vi "TwoBallAuton.vi"(11 "Intake Suck at Beginning?":bool) -> ()   [LabVIEW 2013]
uses:
  <vilib>/Rock Robotics/WPI/SafetyOutput/WPI_SafetyOutputConfigMenu.ctl
  <vilib>/Rock Robotics/WPI/Solenoid/WPI_SolenoidValue.ctl
  <vilib>/Rock Robotics/WPI/RobotDrive/WPI_RobotDriveGetSetRefNum.vi
  <vilib>/Rock Robotics/WPI/Solenoid/WPI_SolenoidSetEnum.vi
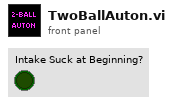
[diagram p1: front panel]
types:
  T1 = typedef "WPI_SafetyOutputConfigMenu.ctl" = enum16{"Enable", "Disable"}
  T2 = typedef "WPI_RobotDriveDevRef.ctl" = cluster{"DevStatus":errorcluster, "Motors[]":T3[], "Square Inputs":bool, "Max Output":dbl, "Isochronous":bool}
  T3 = typedef "WPI_MotorControlDeviceRef.ctl" = cluster{"DeviceStatus":errorcluster, "Type":enum16{"PWM", "CAN"}, "PWM":cluster{"Digital Module":T4, "PWM Channel":T5, "DeadBand":T6}, "CAN":cluster{"Device Number":u8, "Control Mode":T7, "Semaphore":T8, "Max Vout":dbl}, "Invert":bool, "TransformRef":T9, "InvTransformRef":T9}
  T4 = typedef "FPGA_TypedefDigitalModule.ctl" = enum16{"Digital Module 1", "Digital Module 2"}
  T5 = typedef "FPGA_DIOPWMChannel.ctl" = enum8{"PWM 1", "PWM 2", "PWM 3", "PWM 4", "PWM 5", "PWM 6", "PWM 7", "PWM 8", "PWM 9", "PWM 10", "Invalid"}
  T6 = typedef "WPI_PWMDeadband.ctl" = cluster{"Name":string, "maxPositivePwm":i32, "minPositivePwm":i32, "centerPwm":i32, "maxNegativePwm":i32, "minNegativePwm":i32, "angularRange":u16}
  T7 = typedef "WPI_CANJaguar_ControlMode.ctl" = enum8{"Percent VBus", "Current", "Speed", "Position", "Voltage"}
  T8 = typedef "Semaphore RefNum" = refnum<k1>
  T9 = typedef "WPI_PWMTransform_ConPane.ctl" = refnum<vi>
  T10 = typedef "WPI_DigitalInputDevRef.ctl" = cluster{"DevStatus":errorcluster, "DIO Channel":T11, "Digital Module":T4}
  T11 = typedef "FPGA_DIOChannel.ctl" = enum8{"DIO 1", "DIO 2", "DIO 3", "DIO 4", "DIO 5", "DIO 6", "DIO 7", "DIO 8", "DIO 9", "DIO 10", "DIO 11", "DIO 12", "DIO 13", "DIO 14", "Invalid"}
  T12 = typedef "WPI_SolenoidDevRef.ctl" = cluster{"DevStatus":errorcluster, "Solenoid Module":T13, "Forward Solenoid Channel":T14, "Reverse Solenoid Channel":T14}
  T13 = typedef "FPGA_TypedefSolenoidModule.ctl" = enum16{"Solenoid Module 1", "Solenoid Module 2"}
  T14 = typedef "WPI_SolenoidChannel.ctl" = enum8{"Solenoid 1", "Solenoid 2", "Solenoid 3", "Solenoid 4", "Solenoid 5", "Solenoid 6", "Solenoid 7", "Solenoid 8", "Invalid"}
  T15 = typedef "WPI_EncoderDevRef.ctl" = cluster{"DevStatus":errorcluster, "EncoderIndex":T16, "CounterIndex":T17, "DistancePerCount":dbl, "Decoding Type":T18}
  T16 = typedef "FPGA_EncoderIdx.ctl" = enum8{"Enc 0", "Enc 1", "Enc 2", "Enc 3", "Invalid"}
  T17 = typedef "FPGA_CounterCtrSystemIndex.ctl" = enum8{"Ctr 0", "Ctr 1", "Ctr 2", "Ctr 3", "Ctr 4", "Ctr 5", "Ctr 6", "Ctr 7", "Invalid"}
  T18 = typedef "WPI_EncoderType.ctl" = enum16{"1x", "2x", "4x"}
  T19 = typedef "WPI_SolenoidValue.ctl" = enum16{"Off", "On", "Forward", "Reverse"}
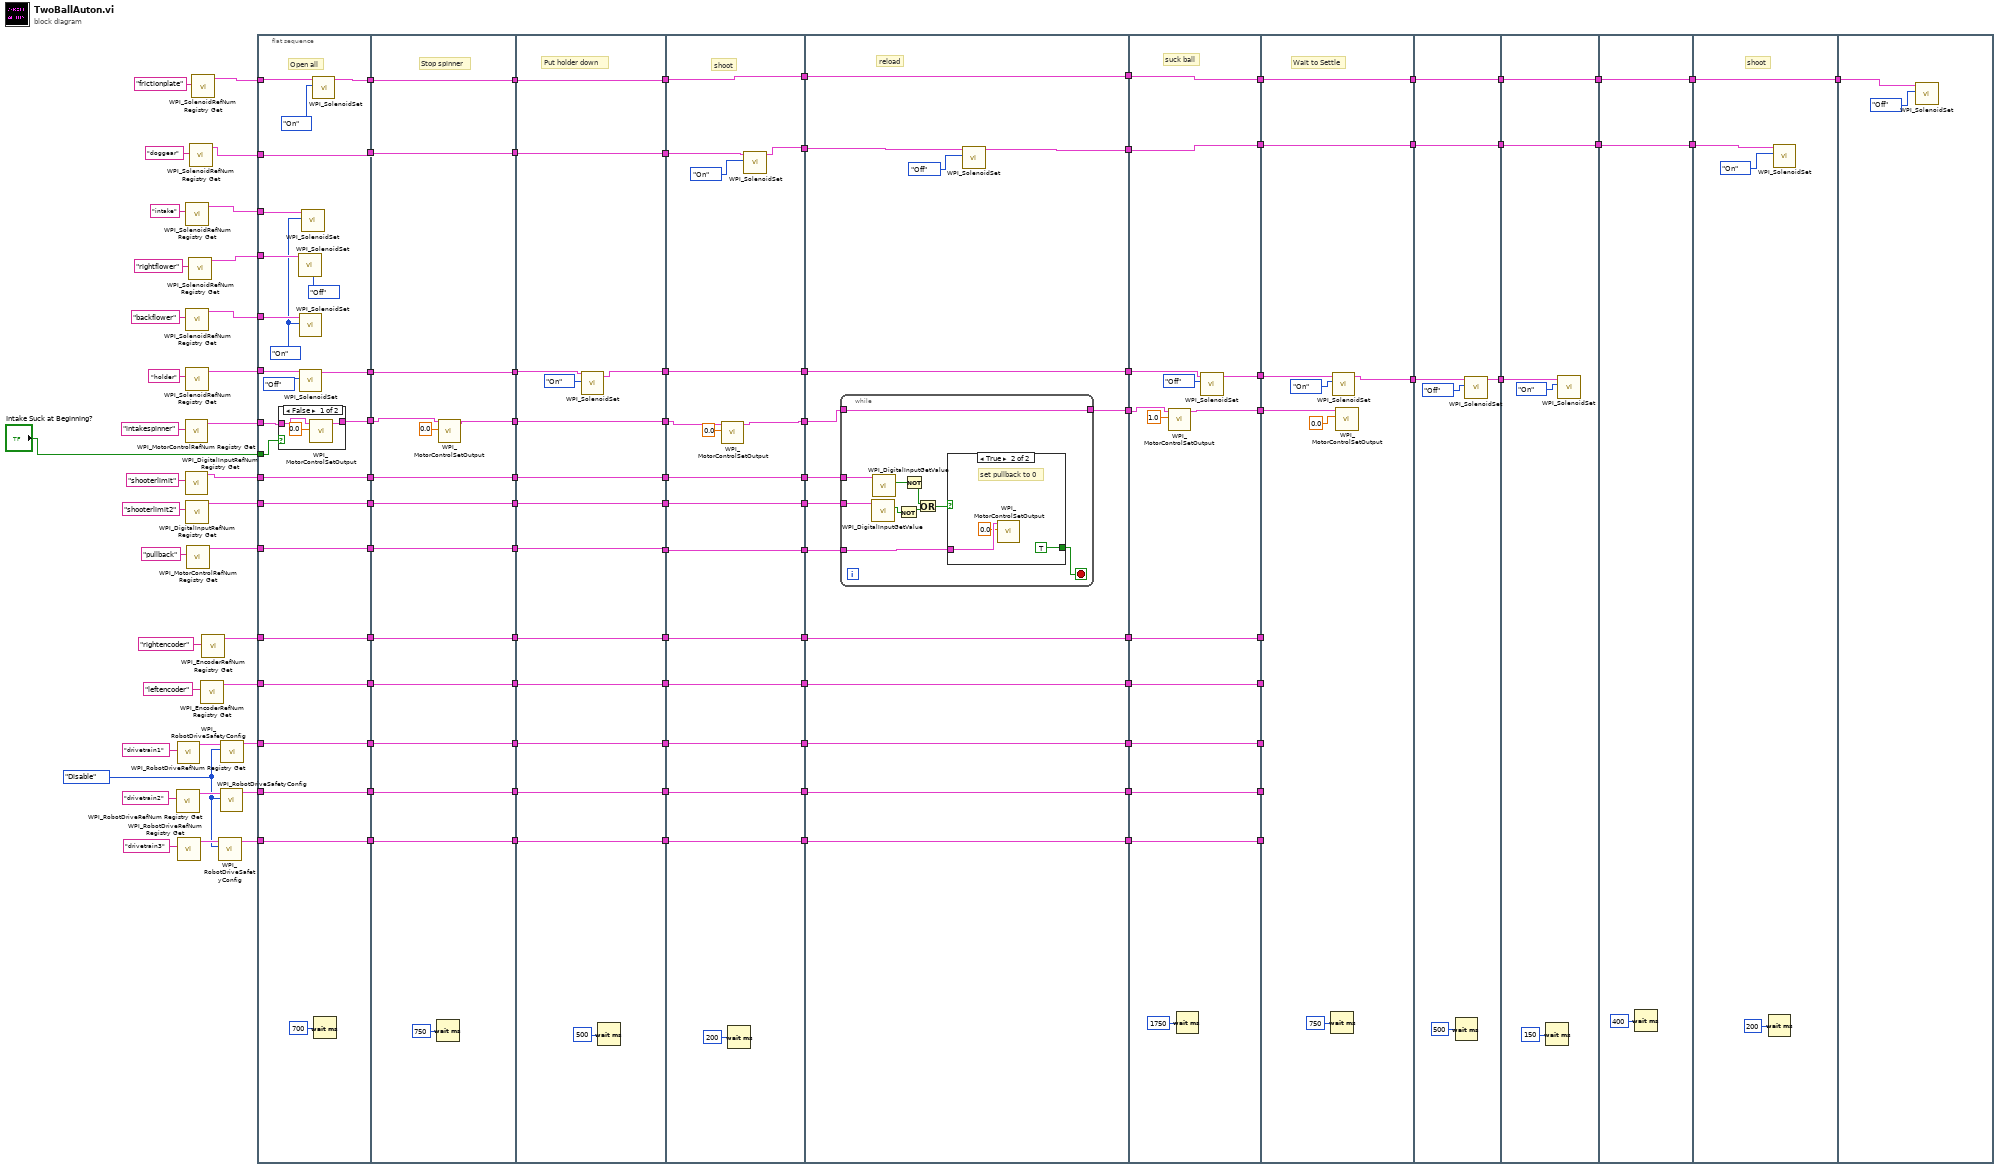
[diagram p0: block diagram]
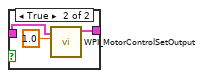
[diagram p2: hidden frame]
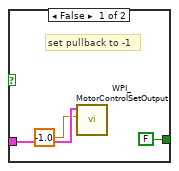
[diagram p3: hidden frame]
diagram:
  w58 = WPI_SafetyOutputConfigMenu."Disable" ("mode")
  n1 = call <vilib>:"WPI_RobotDriveRefNum Registry Get.vi"("refnum name"="drivetrain2") -> ("RobotDriveDevRef"=w60:T2)  [unwired: 9 in, 1 out]
  n2 = call <vilib>:"WPI_RobotDriveRefNum Registry Get.vi"("refnum name"="drivetrain1") -> ("RobotDriveDevRef"=w61:T2)  [unwired: 9 in, 1 out]
  n3 = call <vilib>:"WPI_RobotDriveRefNum Registry Get.vi"("refnum name"="drivetrain3") -> ("RobotDriveDevRef"=w59:T2)  [unwired: 9 in, 1 out]
  n4 = call <vilib>:"WPI_MotorControlRefNum Registry Get.vi"("refnum name"="intakespinner") -> ("MotorControlDevRef"=w71:T3)  [unwired: 9 in, 1 out]
  n5 = call <vilib>:"WPI_DigitalInputRefNum Registry Get.vi"("refnum name"="shooterlimit") -> ("DigitalInputDevRef"=w69:T10)  [unwired: 9 in, 1 out]
  n6 = call <vilib>:"WPI_SolenoidRefNum Registry Get.vi"("refnum name"="intake") -> ("SolenoidDevRef"=w75:T12)  [unwired: 9 in, 1 out]
  n7 = call <vilib>:"WPI_SolenoidRefNum Registry Get.vi"("refnum name"="backflower") -> ("SolenoidDevRef"=w73:T12)  [unwired: 9 in, 1 out]
  n8 = call <vilib>:"WPI_SolenoidRefNum Registry Get.vi"("refnum name"="holder") -> ("SolenoidDevRef"=w39:T12)  [unwired: 9 in, 1 out]
  n9 = call <vilib>:"WPI_DigitalInputRefNum Registry Get.vi"("refnum name"="shooterlimit2") -> ("DigitalInputDevRef"=w43:T10)  [unwired: 9 in, 1 out]
  n10 = call <vilib>:"WPI_MotorControlRefNum Registry Get.vi"("refnum name"="pullback") -> ("MotorControlDevRef"=w67:T3)  [unwired: 9 in, 1 out]
  n11 = call <vilib>:"WPI_SolenoidRefNum Registry Get.vi"("refnum name"="rightflower") -> ("SolenoidDevRef"=w74:T12)  [unwired: 9 in, 1 out]
  n12 = call <vilib>:"WPI_SolenoidRefNum Registry Get.vi"("refnum name"="doggear") -> ("SolenoidDevRef"=w79:T12)  [unwired: 9 in, 1 out]
  n13 = call <vilib>:"WPI_SolenoidRefNum Registry Get.vi"("refnum name"="frictionplate") -> ("SolenoidDevRef"=w50:T12)  [unwired: 9 in, 1 out]
  n14 = call <vilib>:"WPI_EncoderRefNum Registry Get.vi"("refnum name"="leftencoder") -> ("EncoderDevRef"=w56:T15)  [unwired: 9 in, 1 out]
  n15 = call <vilib>:"WPI_EncoderRefNum Registry Get.vi"("refnum name"="rightencoder") -> ("EncoderDevRef"=w57:T15)  [unwired: 9 in, 1 out]
  n16 = call <vilib>:"WPI_RobotDriveSafetyConfig.vi"("mode"=w58, "RobotDriveDevRef"=w59) -> ("RobotDriveDevRef"=w53:T2)  [unwired: 8 in, 1 out]
  n17 = call <vilib>:"WPI_RobotDriveSafetyConfig.vi"("mode"=w58, "RobotDriveDevRef"=w60) -> ("RobotDriveDevRef"=w54:T2)  [unwired: 8 in, 1 out]
  n18 = call <vilib>:"WPI_RobotDriveSafetyConfig.vi"("mode"=w58, "RobotDriveDevRef"=w61) -> ("RobotDriveDevRef"=w55:T2)  [unwired: 8 in, 1 out]
  n19 = flat-sequence {
    tunnel: w79 -> [w136]
    tunnel: [w136] -> w34
    tunnel: w75 -> [w135]
    tunnel: w74 -> [w134]
    tunnel: w73 -> [w133]
    tunnel: w71 -> [w131]
    tunnel: [w130] -> w33
    tunnel: w69 -> [w129]
    tunnel: [w129] -> w32
    tunnel: w67 -> [w128]
    tunnel: [w128] -> w31
    tunnel: [w127] -> w30
    tunnel: w57 -> [w127]
    tunnel: [w126] -> w29
    tunnel: w56 -> [w126]
    tunnel: [w125] -> w28
    tunnel: w55 -> [w125]
    tunnel: [w124] -> w27
    tunnel: w54 -> [w124]
    tunnel: [w123] -> w26
    tunnel: w53 -> [w123]
    tunnel: "Intake Suck at Beginning?" -> [w120]
    tunnel: w50 -> [w118]
    tunnel: [w117] -> w25
    tunnel: w43 -> [w116]
    tunnel: [w116] -> w24
    tunnel: w39 -> [w115]
    tunnel: [w113] -> w23
    tunnel: w34 -> [w157]
    tunnel: [w157] -> w22
    tunnel: w33 -> [w145]
    tunnel: w32 -> [w156]
    tunnel: [w156] -> w21
    tunnel: w31 -> [w155]
    tunnel: [w155] -> w20
    tunnel: w30 -> [w154]
    tunnel: [w154] -> w19
    tunnel: w29 -> [w153]
    tunnel: [w153] -> w18
    tunnel: w28 -> [w152]
    tunnel: [w152] -> w17
    tunnel: w27 -> [w151]
    tunnel: [w151] -> w16
    tunnel: w26 -> [w150]
    tunnel: [w150] -> w15
    tunnel: w25 -> [w149]
    tunnel: [w149] -> w14
    tunnel: w24 -> [w148]
    tunnel: [w148] -> w13
    tunnel: w23 -> [w147]
    tunnel: [w147] -> w12
    tunnel: [w144] -> w11
    tunnel: [w159] -> w112
    tunnel: [w171] -> w111
    tunnel: [w170] -> w110
    tunnel: [w169] -> w109
    tunnel: [w168] -> w108
    tunnel: [w167] -> w107
    tunnel: [w166] -> w106
    tunnel: [w165] -> w105
    tunnel: [w164] -> w104
    tunnel: [w163] -> w47
    tunnel: [w162] -> w42
    tunnel: [w160] -> w38
    tunnel: w22 -> [w169]
    tunnel: w21 -> [w171]
    tunnel: w20 -> [w170]
    tunnel: w19 -> [w167]
    tunnel: w18 -> [w168]
    tunnel: w17 -> [w166]
    tunnel: w16 -> [w165]
    tunnel: w15 -> [w164]
    tunnel: w14 -> [w163]
    tunnel: w13 -> [w162]
    tunnel: w12 -> [w158]
    tunnel: w11 -> [w159]
    tunnel: w112 -> [w187]
    tunnel: [w186] -> w103
    tunnel: w111 -> [w189]
    tunnel: [w189] -> w102
    tunnel: w110 -> [w188]
    tunnel: [w188] -> w101
    tunnel: [w182] -> w100
    tunnel: w109 -> [w181]
    tunnel: [w180] -> w99
    tunnel: w108 -> [w180]
    tunnel: [w179] -> w98
    tunnel: w107 -> [w179]
    tunnel: [w178] -> w97
    tunnel: w106 -> [w178]
    tunnel: [w177] -> w96
    tunnel: w105 -> [w177]
    tunnel: [w176] -> w95
    tunnel: w104 -> [w176]
    tunnel: w47 -> [w175]
    tunnel: [w175] -> w46
    tunnel: w42 -> [w174]
    tunnel: [w174] -> w41
    tunnel: w38 -> [w173]
    tunnel: [w173] -> w37
    tunnel: w103 -> [w201]
    tunnel: w102 -> [w204]
    tunnel: w101 -> [w203]
    tunnel: [w202] -> w93
    tunnel: [w199] -> w94
    tunnel: w100 -> [w198]
    tunnel: [w197] -> w92
    tunnel: w99 -> [w197]
    tunnel: [w196] -> w91
    tunnel: w98 -> [w196]
    tunnel: [w195] -> w90
    tunnel: w97 -> [w195]
    tunnel: [w194] -> w89
    tunnel: w96 -> [w194]
    tunnel: [w193] -> w88
    tunnel: w95 -> [w193]
    tunnel: w46 -> [w192]
    tunnel: [w192] -> w45
    tunnel: w41 -> [w191]
    tunnel: w37 -> [w190]
    tunnel: [w190] -> w36
    tunnel: [w234] -> w81
    tunnel: [w230] -> w82
    tunnel: w94 -> [w234]
    tunnel: w93 -> [w231]
    tunnel: w92 -> [w228]
    tunnel: w91 -> [w229]
    tunnel: [w229] -> w83
    tunnel: [w228] -> w84
    tunnel: [w227] -> w85
    tunnel: w90 -> [w227]
    tunnel: [w226] -> w86
    tunnel: w89 -> [w226]
    tunnel: [w225] -> w87
    tunnel: w88 -> [w225]
    tunnel: [w224] -> w49
    tunnel: w45 -> [w224]
    tunnel: w36 -> [w222]
    tunnel: [w221] -> w35
    tunnel: [w242] -> w10
    tunnel: w87 -> [_]
    tunnel: w86 -> [_]
    tunnel: w85 -> [_]
    tunnel: w84 -> [_]
    tunnel: w83 -> [_]
    tunnel: w82 -> [w239]
    tunnel: w81 -> [w242]
    tunnel: w49 -> [w238]
    tunnel: [w238] -> w9
    tunnel: w35 -> [w237]
    tunnel: [w235] -> w6
    tunnel: w10 -> [w248]
    tunnel: [w248] -> w8
    tunnel: w9 -> [w247]
    tunnel: [w247] -> w7
    tunnel: w6 -> [w245]
    tunnel: [w244] -> w5
    tunnel: w8 -> [w253]
    tunnel: [w253] -> w4
    tunnel: w7 -> [w252]
    tunnel: [w252] -> w2
    tunnel: w5 -> [w250]
    tunnel: w4 -> [w256]
    tunnel: [w256] -> w3
    tunnel: w2 -> [w255]
    tunnel: [w255] -> w1
    tunnel: w3 -> [w258]
    tunnel: w1 -> [w257]
    tunnel: [w257] -> w48
    tunnel: w48 -> [w261]
    frame #0 {
      w122 = WPI_SolenoidValue."On" ("Value")
      # "Open all"
      n20 = case shown="False" w120 {
        tunnel: w131 -> [w138 w142]
        tunnel: [w137 w140] -> w130
        frame False {
          n21 = call <vilib>:"WPI_MotorControlSetOutput.vi"("Output"=0.0, "MotorControlDevRef"=w138) -> ("MotorControlDevRef"=w137:T3)  [unwired: 7 in, 2 out]
        }
        frame True {
          n22 = call <vilib>:"WPI_MotorControlSetOutput.vi"("Output"=1.0, "MotorControlDevRef"=w142) -> ("MotorControlDevRef"=w140:T3)  [unwired: 7 in, 2 out]
        }
      }
      n23 = call-poly <vilib>:"WPI_SolenoidSet.vi"("Value"=WPI_SolenoidValue."Off", "SolenoidDevRef"=w134) -> ()  [unwired: 8 in, 2 out]
      n24 = call-poly <vilib>:"WPI_SolenoidSet.vi"("Value"=w122, "SolenoidDevRef"=w133) -> ()  [unwired: 8 in, 2 out]
      n25 = call-poly <vilib>:"WPI_SolenoidSet.vi"("Value"=WPI_SolenoidValue."Off", "SolenoidDevRef"=w115) -> ("SolenoidDevRef"=w113:T12)  [unwired: 8 in, 1 out]
      n26 = call-poly <vilib>:"WPI_SolenoidSet.vi"("Value"=w122, "SolenoidDevRef"=w135) -> ()  [unwired: 8 in, 2 out]
      n27 = call-poly <vilib>:"WPI_SolenoidSet.vi"("Value"=WPI_SolenoidValue."On", "SolenoidDevRef"=w118) -> ("SolenoidDevRef"=w117:T12)  [unwired: 8 in, 1 out]
      n28 = Wait (ms)(milliseconds to wait=u32 700) -> ()  [unwired: 1 out]
    }
    frame #1 {
      # "Stop spinner"
      n29 = Wait (ms)(milliseconds to wait=u32 750) -> ()  [unwired: 1 out]
      n30 = call <vilib>:"WPI_MotorControlSetOutput.vi"("Output"=0.0, "MotorControlDevRef"=w145) -> ("MotorControlDevRef"=w144:T3)  [unwired: 7 in, 2 out]
    }
    frame #2 {
      # "Put holder down"
      n31 = call-poly <vilib>:"WPI_SolenoidSet.vi"("Value"=WPI_SolenoidValue."On", "SolenoidDevRef"=w158) -> ("SolenoidDevRef"=w160:T12)  [unwired: 8 in, 1 out]
      n32 = Wait (ms)(milliseconds to wait=u32 500) -> ()  [unwired: 1 out]
    }
    frame #3 {
      # "shoot"
      n33 = call <vilib>:"WPI_MotorControlSetOutput.vi"("Output"=0.0, "MotorControlDevRef"=w187) -> ("MotorControlDevRef"=w186:T3)  [unwired: 7 in, 2 out]
      n34 = Wait (ms)(milliseconds to wait=u32 200) -> ()  [unwired: 1 out]
      n35 = call-poly <vilib>:"WPI_SolenoidSet.vi"("Value"=WPI_SolenoidValue."On", "SolenoidDevRef"=w181) -> ("SolenoidDevRef"=w182:T12)  [unwired: 8 in, 1 out]
    }
    frame #4 {
      # "reload"
      n36 = while {
        tunnel: w204 -> [w214]
        tunnel: w203 -> [w212]
        tunnel: [w210] -> w202
        tunnel: w201 -> [w210]
        tunnel: w191 -> [w209]
        stop <- w211 stop-if-true
        n37 = call <vilib>:"WPI_DigitalInputGetValue.vi"("DigitalInputDevRef"=w209) -> ("Value"=w205:bool)  [unwired: 8 in, 2 out]
        n38 = call <vilib>:"WPI_DigitalInputGetValue.vi"("DigitalInputDevRef"=w214) -> ("Value"=w213:bool)  [unwired: 8 in, 2 out]
        n39 = Not(x=w205) -> (.not. x?=w206:bool)
        n40 = Not(x=w213) -> (.not. x?=w208:bool)
        n41 = Or(x=w208, y=w206) -> (x .or. y?=w207:bool)
        n42 = case shown="True" w207 {
          tunnel: w212 -> [w217 w220]
          tunnel: [FALSE TRUE] -> w211
          frame False {
            # "set pullback to -1"
            n43 = call <vilib>:"WPI_MotorControlSetOutput.vi"("Output"=-1.0, "MotorControlDevRef"=w217) -> ()  [unwired: 7 in, 3 out]
          }
          frame True {
            # "set pullback to 0"
            n44 = call <vilib>:"WPI_MotorControlSetOutput.vi"("Output"=0.0, "MotorControlDevRef"=w220) -> ()  [unwired: 7 in, 3 out]
          }
        }
      }
      n45 = call-poly <vilib>:"WPI_SolenoidSet.vi"("Value"=WPI_SolenoidValue."Off", "SolenoidDevRef"=w198) -> ("SolenoidDevRef"=w199:T12)  [unwired: 8 in, 1 out]
    }
    frame #5 {
      # "suck ball"
      n46 = call <vilib>:"WPI_MotorControlSetOutput.vi"("Output"=1.0, "MotorControlDevRef"=w231) -> ("MotorControlDevRef"=w230:T3)  [unwired: 7 in, 2 out]
      n47 = Wait (ms)(milliseconds to wait=u32 1750) -> ()  [unwired: 1 out]
      n48 = call-poly <vilib>:"WPI_SolenoidSet.vi"("Value"=WPI_SolenoidValue."Off", "SolenoidDevRef"=w222) -> ("SolenoidDevRef"=w221:T12)  [unwired: 8 in, 1 out]
    }
    frame #6 {
      # "Wait to Settle"
      n49 = Wait (ms)(milliseconds to wait=u32 750) -> ()  [unwired: 1 out]
      n50 = call-poly <vilib>:"WPI_SolenoidSet.vi"("Value"=WPI_SolenoidValue."On", "SolenoidDevRef"=w237) -> ("SolenoidDevRef"=w235:T12)  [unwired: 8 in, 1 out]
      n51 = call <vilib>:"WPI_MotorControlSetOutput.vi"("Output"=0.0, "MotorControlDevRef"=w239) -> ()  [unwired: 7 in, 3 out]
    }
    frame #7 {
      n52 = Wait (ms)(milliseconds to wait=u32 500) -> ()  [unwired: 1 out]
      n53 = call-poly <vilib>:"WPI_SolenoidSet.vi"("Value"=WPI_SolenoidValue."Off", "SolenoidDevRef"=w245) -> ("SolenoidDevRef"=w244:T12)  [unwired: 8 in, 1 out]
    }
    frame #8 {
      n54 = Wait (ms)(milliseconds to wait=u32 150) -> ()  [unwired: 1 out]
      n55 = call-poly <vilib>:"WPI_SolenoidSet.vi"("Value"=WPI_SolenoidValue."On", "SolenoidDevRef"=w250) -> ()  [unwired: 8 in, 2 out]
    }
    frame #9 {
      n56 = Wait (ms)(milliseconds to wait=u32 400) -> ()  [unwired: 1 out]
    }
    frame #10 {
      # "shoot"
      n57 = Wait (ms)(milliseconds to wait=u32 200) -> ()  [unwired: 1 out]
      n58 = call-poly <vilib>:"WPI_SolenoidSet.vi"("Value"=WPI_SolenoidValue."On", "SolenoidDevRef"=w258) -> ()  [unwired: 8 in, 2 out]
    }
    frame #11 {
      n59 = call-poly <vilib>:"WPI_SolenoidSet.vi"("Value"=WPI_SolenoidValue."Off", "SolenoidDevRef"=w261) -> ()  [unwired: 8 in, 2 out]
    }
  }
